vi "ClearClassMutationHistory.vi"() -> ()   [LabVIEW 2020]
uses:
  <vilib>/Utility/EditLVLibs/Edit LVLibs.lvlib
panel:
  in  "Classes":i32[](listbox) caption="Classes with Mutation History"
  in  "Clear History":bool
  out "Project Name":string
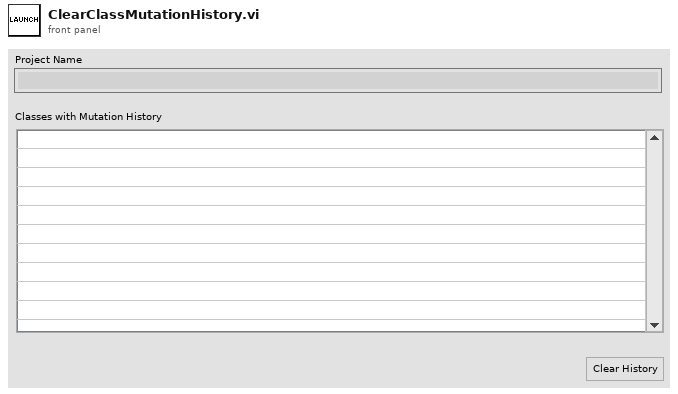
[diagram p1: front panel]
types:
  T1 = enum32{"Invalid", "Standard", "Closed", "Hidden", "Minimized", "Maximized"}
  T2 = typedef "Edit LVLibs.lvlib/Mutation History.ctl" = T3[]
  T3 = typedef "Edit LVLibs.lvlib/Mutation Record.ctl" = cluster{"Library Version":T4, "Old Name Index":u8, "Class Default Data":variant, "Cluster Order Map":u32[], "Parent Name":string, "Parent Path":path, "LabVIEW Version":u32, "User Comments":string, "Mutation Flags":u8, "Parent Old Name Index":u8, "Parent Levels Added":u16, "Parent Levels Removed":u16}
  T4 = typedef "Edit LVLibs.lvlib/LibVersion.ctl" = cluster{"Major":u16, "Minor":u16, "Fix":u16, "Build":u16}
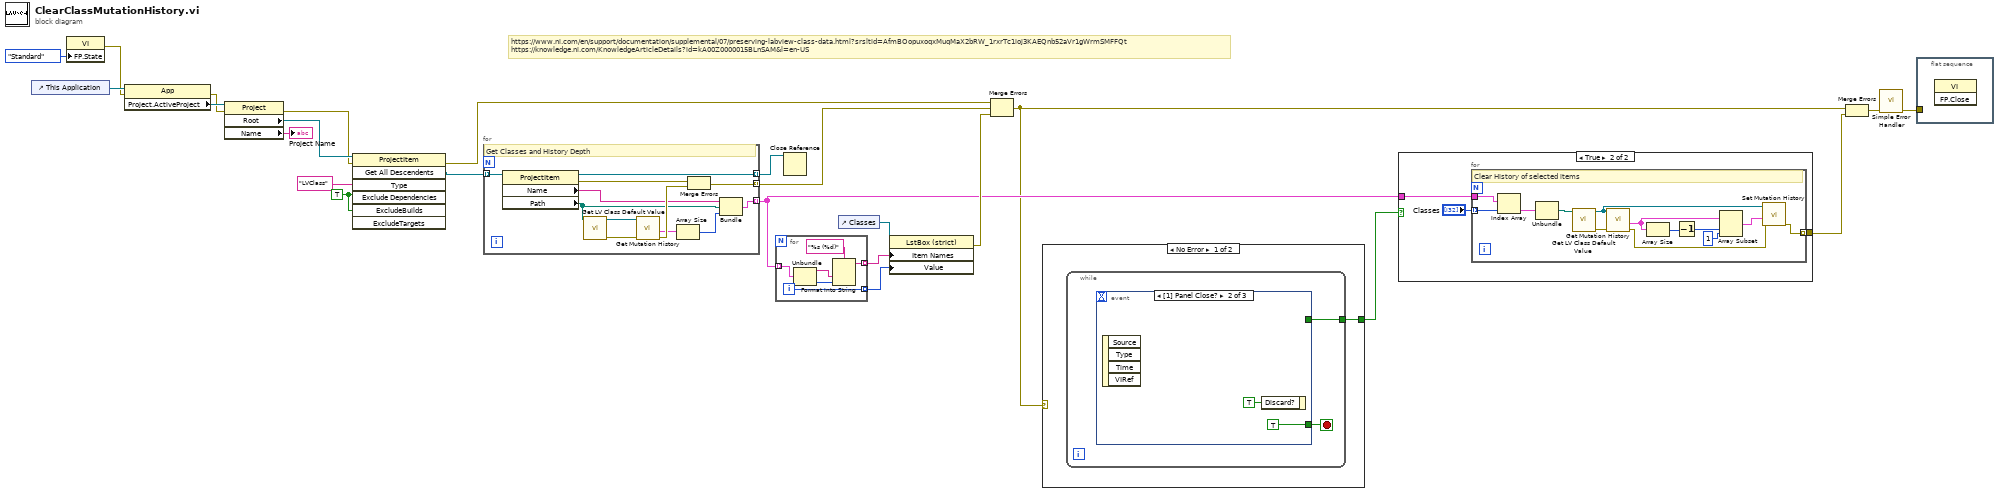
[diagram p0: block diagram]
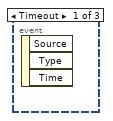
[diagram p2: hidden frame]
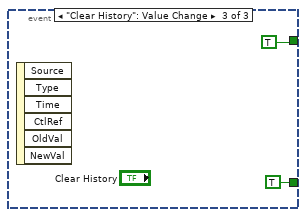
[diagram p3: hidden frame]
diagram:
  w18 = TRUE ("ExcludeDependencies")
  # "https://www.ni.com/en/support/documentation/supplemental/07/preserving-labview-class-data.html?srsltid=AfmBOopuxoqxMuqMaX2bRW_1rxrTc1ioj3KAEQnb52aVr1gWrmSMFFQt\nhttps://knowledge.ni.com/KnowledgeArticleDetails?id=kA00Z0000015BLnSAM&l=en-US"
  n1 = control-ref of="This Application"() -> (w24:refnum<vi>)
  n2 = property class="VI"("FP.State"=T1."Standard" ("Front Panel Window:State")) -> (error out=w22:errorcluster)  [unwired: 2 in, 1 out]
  n3 = property class="App"(reference=w24, error in=w22) -> (error out=w12:errorcluster, "Project.ActiveProject"=w21:refnum<vi>)  [unwired: 1 out]
  n4 = property class="Project"(reference=w21, error in=w12) -> (error out=w11:errorcluster, "Root"=w20:refnum<vi>, "Name"=→"Project Name":string)  [unwired: 1 out]
  n5 = invoke class="ProjectItem" method="Get All Descendents"(reference=w20, error in=w11, "Type"="LVClass", "Exclude Dependencies"=w18, "ExcludeBuilds"=w18) -> (error out=w13:errorcluster, "All Descendents"=w17:refnum<vi>[])  [unwired: 2 in, 5 out]
  n6 = for {
    tunnel: w17 -> [w36] mode=indexing
    tunnel: [w34] -> w6 mode=indexing
    tunnel: [w33] -> w16 mode=indexing
    tunnel: [w25] -> w10 mode=indexing
    # "Get Classes and History Depth"
    n7 = property class="ProjectItem"(reference=w36) -> (reference out=w25:refnum<vi>, error out=w35:errorcluster, "Name"=w26:string, "Path"=w27:path)  [unwired: 1 in]
    n8 = call <vilib>:"Get LV Class Default Value.vi"("class path"=w27) -> ("error out"=w30:errorcluster, "object"=w29:refnum<class>)  [unwired: 9 in]
    n9 = call <vilib>:"Get Mutation History.vi"("error in"=w30, "Input object"=w29) -> ("error out"=w32:errorcluster, "Mutation History"=w31:T2)  [unwired: 6 in]
    n10 = Array Size(array=w31) -> (size(s)=w28:i32)
    n11 = Merge Errors(w35, w32) -> (w33:errorcluster)
    n12 = Bundle("Name"=w26, "Path"=w27, w28) -> (w34:cluster{"Name":string, "Path":path, i32})  [unwired: 1 in]
  }
  n13 = for {
    tunnel: w6 -> [w42] mode=indexing
    tunnel: [w40] -> w8 mode=indexing
    tunnel: [w41] -> w1 mode=indexing
    i -> [w41]
    n14 = Unbundle(w42) -> ("Name"=w38:string, w39:i32)  [unwired: 1 out]
    n15 = Format Into String(format string="%s (%d)", w38, w39) -> (resulting string=w40:string)  [unwired: 2 in, 1 out]
  }
  n16 = Close Reference(reference=w10) -> ()  [unwired: 1 in, 1 out]
  n17 = control-ref of="Classes"() -> (w9:refnum<vi>)
  n18 = property class="LstBox (strict)"(reference=w9, "Item Names"=w8, "Value"=w1) -> (error out=w7:errorcluster)  [unwired: 1 in, 1 out]
  n19 = Merge Errors(w13, w16, w7) -> (w3:errorcluster)
  n20 = case shown="No Error" w3 {
    tunnel: [w43 _] -> w2
    frame No Error {
      n21 = while {
        tunnel: [w44] -> w43
        stop <- w45 stop-if-true
        n22 = event shown="[1] Panel Close?" {
          selector: _ -> [_ _ _]
          dyn-events: _ -> [_ _ _]
          timeout: _ -> [_ _ _]
          tunnel: [_ TRUE ("Discard?") TRUE ("Discard?")] -> w45
          tunnel: [_ _ TRUE] -> w44
          event Timeout {
            n23 = event-data() -> ()  [unwired: 1 in, 3 out]
          }
          event Panel Close? {
            n24 = event-data() -> ()  [unwired: 1 in, 4 out]
            n25 = event-data("Discard?"=TRUE) -> ()  [unwired: 1 in, 1 out]
          }
          event "Clear History": Value Change {
            n26 = event-data() -> ()  [unwired: 1 in, 6 out]
          }
        }
      }
    }
    frame Error {
    }
  }
  n27 = case shown="True" w2 {
    tunnel: w6 -> [_ w51]
    tunnel: [_ w50] -> w4
    frame False {
    }
    frame True {
      n28 = for {
        tunnel: "Classes" -> [w58] mode=indexing
        tunnel: w51 -> [w57]
        tunnel: [w53] -> w50 mode=indexing
        # "Clear History of selected items"
        n29 = Index Array(array=w57, index=w58) -> (element=w56:cluster{"Name":string, "Path":path, i32})
        n30 = Unbundle(w56) -> ("Path"=w55:path)  [unwired: 2 out]
        n31 = call <vilib>:"Get LV Class Default Value.vi"("class path"=w55) -> ("error out"=w54:errorcluster, "object"=w60:refnum<class>)  [unwired: 9 in]
        n32 = call <vilib>:"Get Mutation History.vi"("error in"=w54, "Input object"=w60) -> ("Mutation History"=w61:T2)  [unwired: 6 in, 1 out]
        n33 = Array Size(array=w61) -> (size(s)=w59:i32)
        n34 = Decrement(x=w59) -> (x-1=w62:i32)
        n35 = Array Subset(array=w61, index=w62, length=1) -> (w64:T2)
        n36 = call <vilib>:"Set Mutation History.vi"("error in"=w54, "Mutation History"=w64, "Input object"=w60) -> ("error out"=w53:errorcluster)  [unwired: 8 in]
      }
    }
  }
  n37 = Merge Errors(w3, w4) -> (w5:errorcluster)
  n38 = call <vilib>:"Simple Error Handler.vi"("error in (no error)"=w5) -> ("error out"=w15:errorcluster)  [unwired: 4 in, 4 out]
  n39 = flat-sequence {
    tunnel: w15 -> [_]
    frame #0 {
      n40 = invoke class="VI" method="FP.Close"() -> ()  [unwired: 3 in, 3 out]
    }
  }
